vi "Derivative balance.vi"() -> (3 "Motor Power":dbl)   [LabVIEW 2020]
uses:
  Robot Global Data.vi
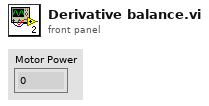
[diagram p1: front panel]
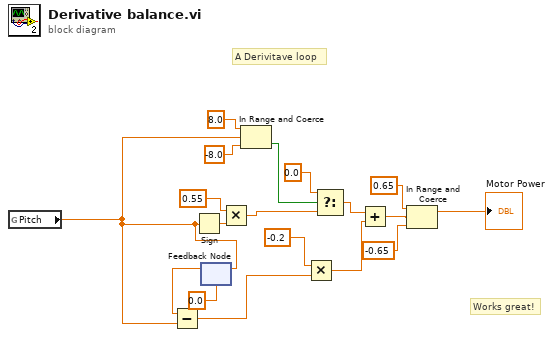
[diagram p0: block diagram]
diagram:
  # "Works great!"
  # "A Derivitave loop"
  n1 = global read "Robot Global Data.vi" "Pitch"() -> (w1:dbl)
  n2 = Sign(1:w1) -> (0:w5:dbl)
  n3 = feedback-in #1(w1) -> ()
  n4 = feedback #1(0.0) -> (w7:dbl)
  n5 = Subtract(x=w7, y=w1) -> (x-y=w17:dbl)
  n6 = Multiply(x=0.55, y=w5) -> (x*y=w15:dbl)
  n7 = In Range and Coerce(upper limit=8.0, x=w1, lower limit=-8.0) -> (In Range?=w12:bool)  [unwired: 1 out]
  n8 = Multiply(x=-0.2, y=w17) -> (x*y=w8:dbl)
  n9 = Select(t=0.0, s=w12, f=w15) -> (s? t:f=w10:dbl)
  n10 = Add(x=w10, y=w8) -> (x+y=w9:dbl)
  n11 = In Range and Coerce(upper limit=0.65, x=w9, lower limit=-0.65) -> (coerced(x)=→"Motor Power":dbl)  [unwired: 1 out]
